vi "EX5.vi"() -> ()   [LabVIEW 2018]
panel:
  in  "Débit":i32(slide) scale=0.0..10.0
  out "Numeric 2":i64
  out "Tank":dbl(slide) scale=0.0..1100.0
  in  "stop":bool
  in  "Numeric":i32 min=0 max=1000
  in  "Consigne":i32(slide) min=0 max=1100 scale=0.0..1100.0
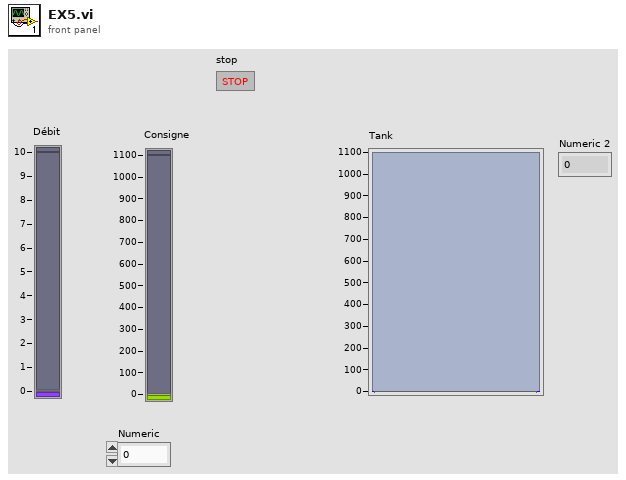
[diagram p1: front panel]
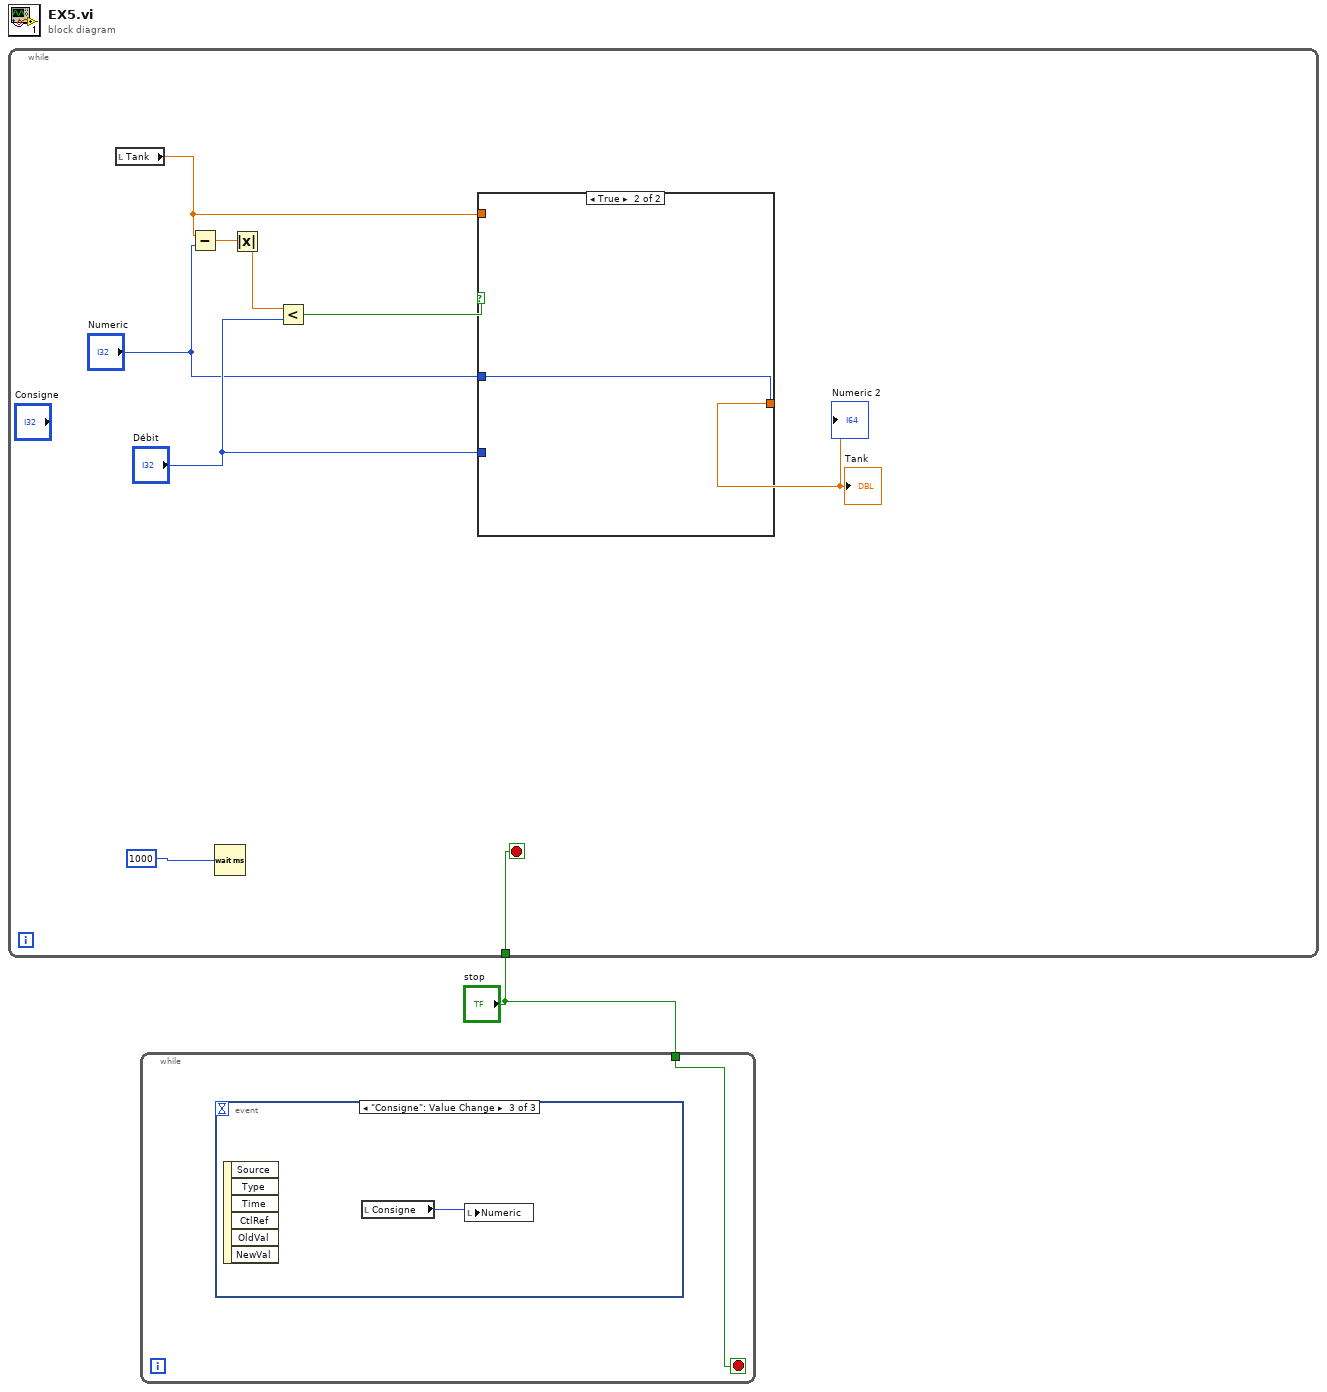
[diagram p0: block diagram]
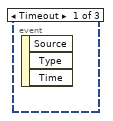
[diagram p2: hidden frame]
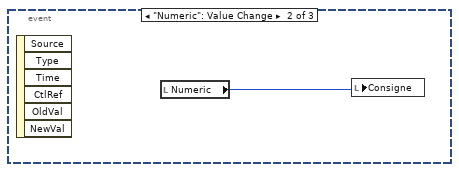
[diagram p3: hidden frame]
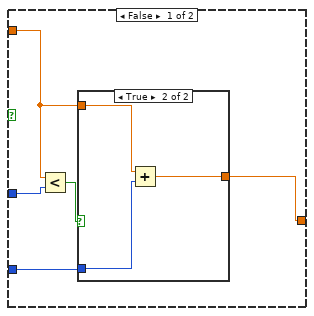
[diagram p4: hidden frame]
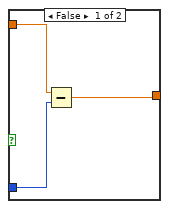
[diagram p5: hidden frame]
diagram:
  n1 = while {
    tunnel: "stop" -> [w2]
    stop <- w2 stop-if-true
    n2 = local read "Tank"() -> (w6:dbl)
    n3 = Subtract(x=w6, y="Numeric") -> (x-y=w9:dbl)
    n4 = Wait (ms)(milliseconds to wait=1000) -> ()  [unwired: 1 out]
    n5 = Absolute Value(x=w9) -> (abs(x)=w8:dbl)
    n6 = Less?(x=w8, y="Débit") -> (x < y?=w7:bool)
    n7 = case shown="True" w7 {
      tunnel: w6 -> [w14 _]
      tunnel: [w12 w22] -> w4
      tunnel: "Débit" -> [w13 _]
      tunnel: "Numeric" -> [w11 w22]
      frame False {
        n8 = Less?(x=w14, y=w11) -> (x < y?=w15:bool)
        n9 = case shown="True" w15 {
          tunnel: w14 -> [w18 w21]
          tunnel: w13 -> [w17 w20]
          tunnel: [w16 w19] -> w12
          frame False {
            n10 = Subtract(x=w18, y=w17) -> (x-y=w16:dbl)
          }
          frame True {
            n11 = Add(x=w21, y=w20) -> (x+y=w19:dbl)
          }
        }
      }
      frame True {
      }
    }
    "Tank" <- w4
    "Numeric 2" <- w4
  }
  n12 = while {
    tunnel: "stop" -> [w23]
    stop <- w23 stop-if-true
    n13 = event shown="[2] \"Consigne\": Value Change" {
      selector: _ -> [_ _ _]
      dyn-events: _ -> [_ _ _]
      timeout: _ -> [_ _ _]
      event Timeout {
        n14 = event-data() -> ()  [unwired: 1 in, 3 out]
      }
      event "Numeric": Value Change {
        n15 = event-data() -> ()  [unwired: 1 in, 6 out]
        n16 = local read "Numeric"() -> (w24:i32)
        n17 = local write "Consigne"(w24) -> ()
      }
      event "Consigne": Value Change {
        n18 = event-data() -> ()  [unwired: 1 in, 6 out]
        n19 = local read "Consigne"() -> (w25:i32)
        n20 = local write "Numeric"(w25) -> ()
      }
    }
  }
